vi "TDMS_writeTable.vi"() -> ()   [LabVIEW 2011]
panel:
  out "error out":errorcluster
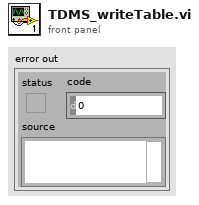
[diagram p1: front panel]
types:
  T1 = enum16{"open", "open or create", "create or replace", "create", "open (read-only)"}
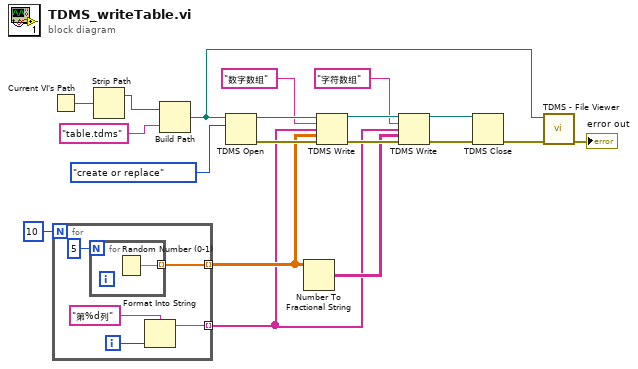
[diagram p0: block diagram]
diagram:
  n1 = Current VI's Path() -> (path=w19:path)
  n2 = for {
    N: 10 -> [_]
    tunnel: [w23] -> w4 mode=indexing
    tunnel: [w22] -> w3 mode=indexing
    i -> [w24]
    n3 = for {
      N: 5 -> [_]
      tunnel: [w25] -> w23 mode=indexing
      n4 = Random Number (0-1)() -> (number: 0 to 1=w25:dbl)
    }
    n5 = Format Into String(format string="第%d列" ("initial string"), w24) -> (resulting string=w22:string)  [unwired: 2 in, 1 out]
  }
  n6 = Strip Path(path=w19) -> (stripped path=w18:path)  [unwired: 1 out]
  n7 = Build Path(base path=w18, name or relative path="table.tdms") -> (appended path=w2:path)
  n8 = TDMS Open(10:T1."create or replace" ("operation (0:open)"), 11:w2) -> (0:w15:errorcluster, 3:w16:refnum<k34>)  [unwired: 4 in]
  n9 = Number To Fractional String(number=w4) -> (F-format string=w5:string[][])  [unwired: 3 in]
  n10 = TDMS Write(0:w16, 5:"数字数组" ("group name in (Untitled)"), 7:w3, 9:w4, 11:w15) -> (4:w13:refnum<k34>, 15:w14:errorcluster)  [unwired: 1 in, 2 out]
  n11 = TDMS Write(0:w13, 5:"字符数组" ("group name in (Untitled)"), 7:w3, 9:w5, 11:w14) -> (4:w12:refnum<k34>, 15:w11:errorcluster)  [unwired: 1 in, 2 out]
  n12 = TDMS Close(8:w11, 11:w12) -> (0:w10:errorcluster)  [unwired: 1 out]
  n13 = call <vilib>:"TDMS - File Viewer.vi"("error in (no error)"=w10, "file path"=w2) -> ("error out"=→"error out":errorcluster)  [unwired: 4 in, 1 out]
